vi "Set View VI Reference.vi"(8 "error in (no error)":errorcluster, 10 "View VI ref":refnum<vi>, 11 "Debug View in":refnum<class "Debug View.lvclass">) -> (0 "error out":errorcluster, 3 "Debug View out":refnum<class "Debug View.lvclass">)   [LabVIEW 2020, in "Debug View.lvclass"]
uses:
  Debug View.lvclass
  Debug View.lvclass/Debug View.ctl
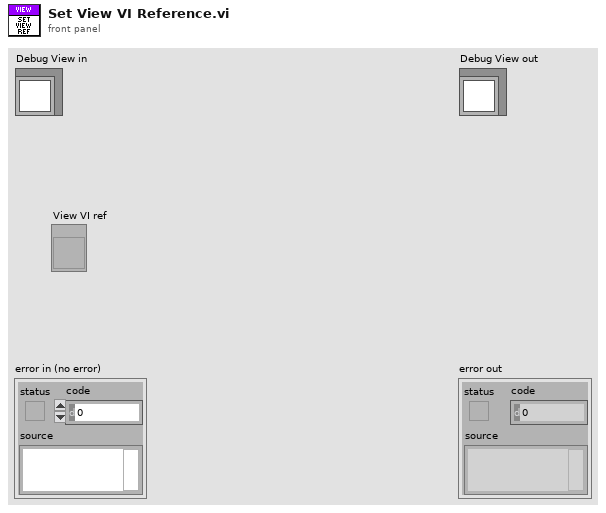
[diagram p1: front panel]
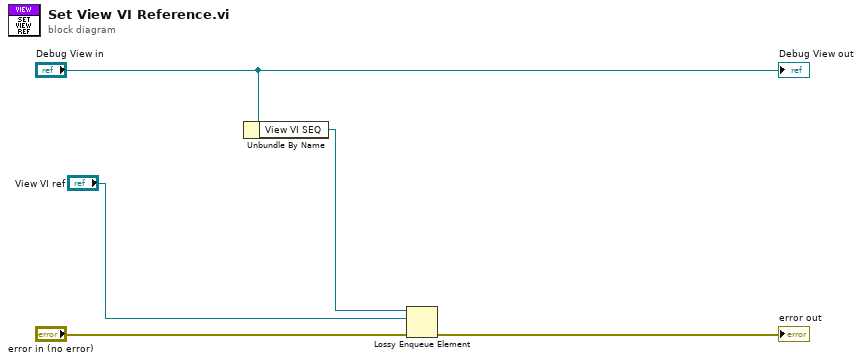
[diagram p0: block diagram]
diagram:
  n1 = Unbundle By Name("Debug View in") -> ("View VI SEQ"=w2:refnum<queue>)
  n2 = Lossy Enqueue Element(queue=w2, element="View VI ref", error in (no error)="error in (no error)") -> (error out=→"error out":errorcluster)  [unwired: 3 out]
  "Debug View out" <- "Debug View in"
